vi "Get Trigger Block List.vi"(8 "error in (no error)":errorcluster, 11 "VISA resource name":refnum<visa-resource-name>) -> (0 "error out":errorcluster, 2 "Trigger Block List":string, 3 "VISA resource name out":refnum<visa-resource-name>)   [LabVIEW 2017, in "Keithley 2450.lvlib"]
doc: "This VI returns the settings for all trigger model building blocks."
uses:
  Keithley 2450.lvlib
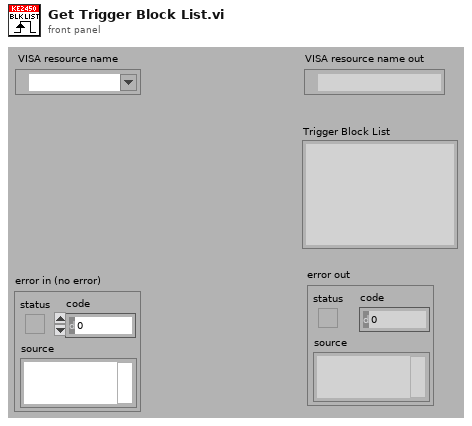
[diagram p1: front panel]
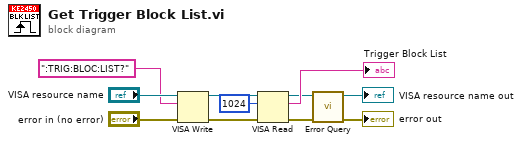
[diagram p0: block diagram]
diagram:
  n1 = VISA Write(VISA resource name="VISA resource name", write buffer=":TRIG:BLOC:LIST?" ("format string"), error in (no error)="error in (no error)") -> (VISA resource name out=w6:refnum<visa-resource-name>, error out=w5:errorcluster)  [unwired: 1 out]
  n2 = VISA Read(VISA resource name=w6, byte count=u32 1024, error in (no error)=w5) -> (VISA resource name out=w4:refnum<visa-resource-name>, read buffer=→"Trigger Block List":string, error out=w2:errorcluster)  [unwired: 1 out]
  n3 = call "Error Query.vi"("error in (no error)"=w2, "VISA resource name"=w4) -> ("error out"=→"error out":errorcluster, "VISA resource name out"=→"VISA resource name out":refnum<visa-resource-name>)  [unwired: 8 out]
